vi "send.vi"(8 "error in (no error)":errorcluster, 10 "Bytes":u8[](array[numeric]), 11 "MOXAIP in":refnum<class "MOXAIP.lvclass">) -> (0 "error out":errorcluster, 3 "MOXAIP out":refnum<class "MOXAIP.lvclass">)   [LabVIEW 2017, in "Serializer.lvlib" / "MOXAIP.lvclass"]
uses:
  MOXAIP.lvclass
  MOXAIP.lvclass/MOXAIP.ctl
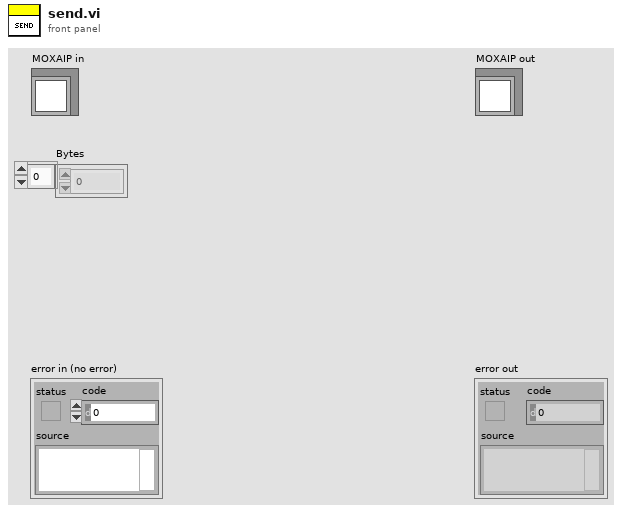
[diagram p1: front panel]
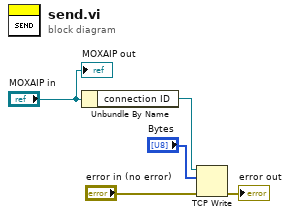
[diagram p0: block diagram]
diagram:
  n1 = Unbundle By Name("MOXAIP in") -> ("connection ID"=w4:refnum<k5>)
  n2 = TCP Write(connection ID=w4, data in="Bytes", error in (no error)="error in (no error)") -> (error out=→"error out":errorcluster)  [unwired: 1 in, 2 out]
  "MOXAIP out" <- "MOXAIP in"
